vi "PWM FPGA test2.vi"() -> ()   [LabVIEW 2013]
uses:
  <vilib>/Platform/TimedLoop/XDataNode/timing_clust.ctl
  <vilib>/Platform/TimedLoop/XDataNode/nitl_modes.ctl
  <vilib>/Platform/TimedLoop/XDataNode/wakeup.ctl
  <vilib>/rvi/Emulation/niFpgaSctlEmulationGetInTimedLoop.vi
  <vilib>/rvi/Emulation/niFpgaEmulationReportErrorSimple.vi
  <vilib>/rvi/Emulation/niFpgaGetClockAttributes.vi
  <vilib>/rvi/Emulation/niFpgaCriticalErrorInLSC.vi
  <vilib>/rvi/eio/common/nirviEmuTemplateMethod_errors.vi
  <vilib>/Platform/TimedLoop/XDataNode/XDataNode.xnode
  <vilib>/eio/EIONode/EIONode.xnode
  <vilib>/Platform/TimedLoop/XDataNode/XDNodeRunTimeDep.lvlib
panel:
  in  "TTL 2":bool
  in  "TTL 3":bool
  in  "TTL 4":bool
  in  "TTL 1":bool
  in  "ISO Out 2":bool
  in  "ISO Out 1":bool
  in  "ISO Out 0":bool
  in  "frequency (periods/tick)":fxp<+,32,0>=0.0007812499534338713
  in  "duty cycle (periods)":fxp<+,16,0>=0.5
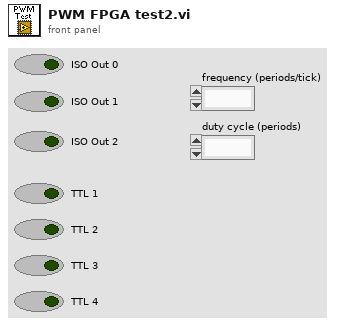
[diagram p1: front panel]
types:
  T1 = typedef "XDNodeRunTimeDep.lvlib/timing_clust.ctl" = cluster{"Expected End [f-1]":u64, "Actual End [f-1]":u64, "Finished Late? [f-1]":bool, "Expected End [i-1]":u64, "Actual End [i-1]":u64, "Finished Late? [i-1]":bool, "Expected Start [i]":u64, "Actual Start [i]":u64, "Expected Start [f]":u64, "Actual Start [f]":u64, "Source Name":string, "Structure Name":string, "Period":i64, "Deadline":i64, "Offset":i64, "Start":i64, "Priority":i32, "Timeout":i32, "Mode":T2, "Wakeup Reason":T3, "Error":errorcluster, "Source Type":string, "Secondary Source Type":string, "Global End Time":u64, "Global Start Time":u64, "Frame Duration":u64, "Iteration Duration":u64, "Assigned CPU":i32, "I/O Scan Engine Mode":u32}
  T2 = typedef "XDNodeRunTimeDep.lvlib/nitl_modes.ctl" = enum32{"No Change", "Process missed periods, maintain original phase", "Discard missed periods, maintain original phase", "Process missed periods, ignore original phase", "Discard missed periods, ignore original phase"}
  T3 = typedef "XDNodeRunTimeDep.lvlib/wakeup.ctl" = enum32{"Normal", "Aborted", "Asynchronous wakeup", "Timing source error", "Timed loop error", "Timeout"}
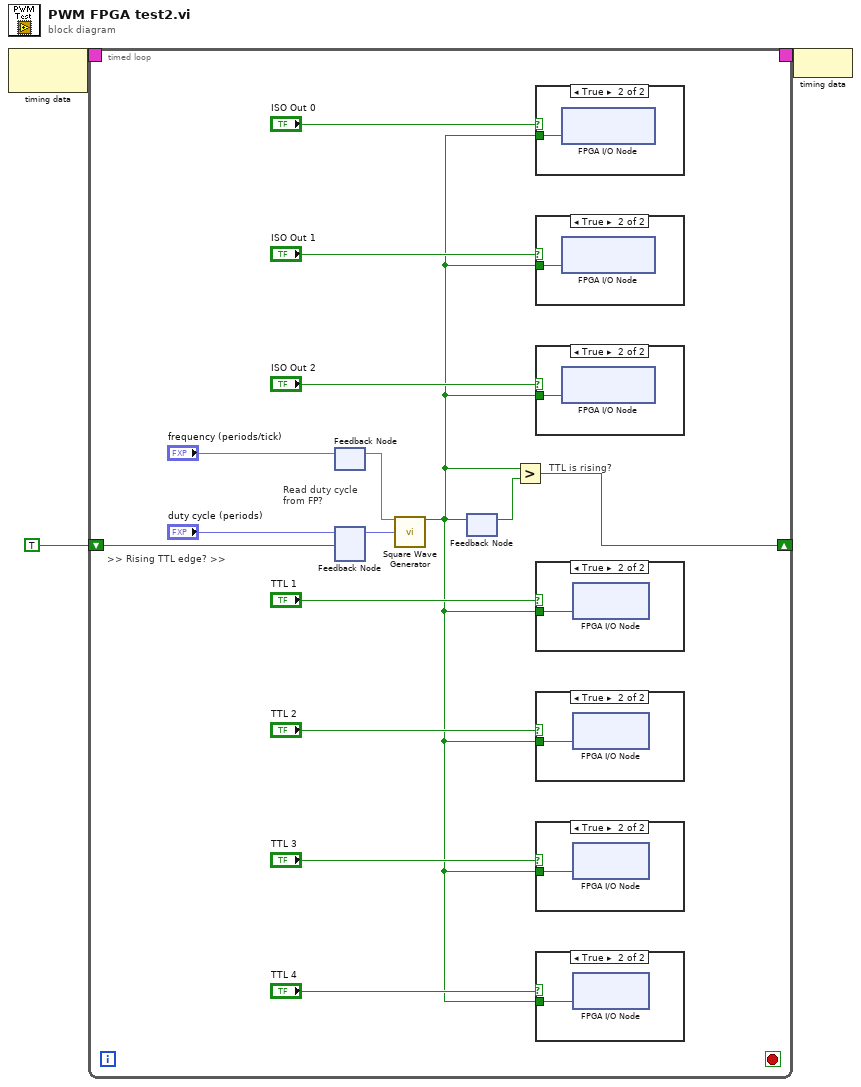
[diagram p0: block diagram]
diagram:
  n1 = node-c288 ("Input Node")() -> (w2:T1)  [unwired: 1 in]
  n2 = timed-loop {
    timing: w2 -> [_]
    timing-out: [_] -> w1
    shift-right: [w4] -> _
    shift-left: TRUE -> [w18]
    stop <- _ stop-if-true
    # "Read duty cycle\nfrom FP?"
    # ">> Rising TTL edge? >>"
    # "TTL is rising?"
    n3 = feedback #1() -> (w15:fxp<+,32,0>)  [unwired: 1 in]
    n4 = feedback-in #1("frequency (periods/tick)") -> ()
    n5 = feedback #2() -> (w14:fxp<+,16,0>)  [unwired: 1 in]
    n6 = feedback-in #2("duty cycle (periods)", w18) -> ()
    n7 = call "Square Wave Generator"("frequency (periods/tick)"=w15, "duty cycle (periods)"=w14) -> ("square wave out"=w5:bool)  [unwired: 13 in]
    n8 = feedback #3() -> (w8:bool)  [unwired: 1 in]
    n9 = feedback-in #3(w5) -> ()
    n10 = Greater?(x=w5, y=w8) -> (0:w4:bool)
    n11 = case shown="True" "ISO Out 0" {
      tunnel: w5 -> [_ w25]
      frame False {
      }
      frame True {
        n12 = xnode "FPGA I/O Node"("ISO Out 0"=w25) -> ()  [unwired: 1 in, 1 out]
      }
    }
    n13 = case shown="True" "ISO Out 1" {
      tunnel: w5 -> [_ w24]
      frame False {
      }
      frame True {
        n14 = xnode "FPGA I/O Node"("ISO Out 1"=w24) -> ()  [unwired: 1 in, 1 out]
      }
    }
    n15 = case shown="True" "ISO Out 2" {
      tunnel: w5 -> [_ w23]
      frame False {
      }
      frame True {
        n16 = xnode "FPGA I/O Node"("ISO Out 2"=w23) -> ()  [unwired: 1 in, 1 out]
      }
    }
    n17 = case shown="True" "TTL 1" {
      tunnel: w5 -> [_ w22]
      frame False {
      }
      frame True {
        n18 = xnode "FPGA I/O Node"("TTL 1"=w22) -> ()  [unwired: 1 in, 1 out]
      }
    }
    n19 = case shown="True" "TTL 2" {
      tunnel: w5 -> [_ w19]
      frame False {
      }
      frame True {
        n20 = xnode "FPGA I/O Node"("TTL 2"=w19) -> ()  [unwired: 1 in, 1 out]
      }
    }
    n21 = case shown="True" "TTL 3" {
      tunnel: w5 -> [_ w20]
      frame False {
      }
      frame True {
        n22 = xnode "FPGA I/O Node"("TTL 3"=w20) -> ()  [unwired: 1 in, 1 out]
      }
    }
    n23 = case shown="True" "TTL 4" {
      tunnel: w5 -> [_ w21]
      frame False {
      }
      frame True {
        n24 = xnode "FPGA I/O Node"("TTL 4"=w21) -> ()  [unwired: 1 in, 1 out]
      }
    }
  }
  n25 = node-c288(w1) -> ()
